vi "cluster to global variables.vi"(11 "Input Variables and Slopes in":T1 {"Height of Sample Box" format="%.2f"; "Reservoir Pressure" format="%.2f"; "Flow Offset" format="%.2f"; "String Pot Offset" format="%.2f"; "Aux 3 Offset" format="%.2f"; "Aux 2 Offset" format="%.2f"; "Aux 1 Offset" format="%.2f"; "Aux 3 Slope" format="%.2f"; "Aux 2 Slope" format="%.2f"; "Aux 1 Slope" format="%.2f"; "Up Hole  Pressure Offset" format="%.2f"; "DH Pressure Offset" format="%.2f"; "DH Pressure Trans Slope" format="%.2f"; "Atmospheric Pressure" format="%.2f"; "Depth to Water Table" format="%.2f"; "Up Hole Pressure Slope" format="%.2f"; "Flow Slope" format="%.2f"; "String Pot Slope" format="%.2f"; "Total Volume" format="%.2f"}) -> ()   [LabVIEW 2016]
uses:
  KPRO_2016 subvis/Control 2.ctl
  KPRO_2016 subvis/Kpro Globals.vi
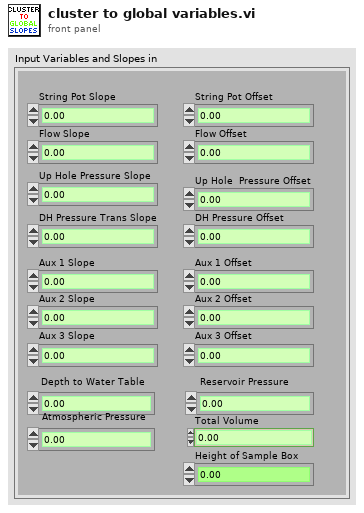
[diagram p1: front panel]
types:
  T1 = typedef "Control 2.ctl" = cluster{"Total Volume":dbl, "String Pot Slope":dbl, "Flow Slope":dbl, "Up Hole Pressure Slope":dbl, "Depth to Water Table":dbl, "Atmospheric Pressure":dbl, "DH Pressure Trans Slope":dbl, "DH Pressure Offset":dbl, "Up Hole  Pressure Offset":dbl, "Aux 1 Slope":dbl, "Aux 2 Slope":dbl, "Aux 3 Slope":dbl, "Aux 1 Offset":dbl, "Aux 2 Offset":dbl, "Aux 3 Offset":dbl, "String Pot Offset":dbl, "Flow Offset":dbl, "Reservoir Pressure":dbl, "Height of Sample Box":dbl}
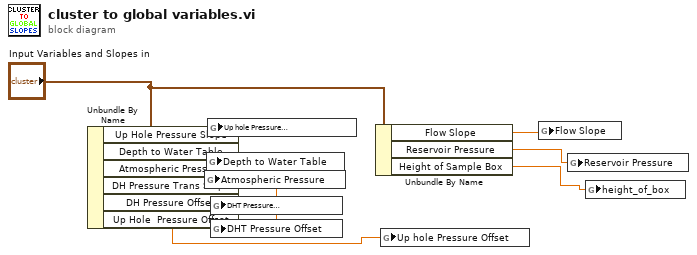
[diagram p0: block diagram]
diagram:
  n1 = Unbundle By Name("Input Variables and Slopes in") -> ("Up Hole Pressure Slope"=w1:dbl, "Depth to Water Table"=w2:dbl, "Atmospheric Pressure"=w3:dbl, "DH Pressure Trans Slope"=w4:dbl, "DH Pressure Offset"=w5:dbl, "Up Hole  Pressure Offset"=w6:dbl)
  n2 = global write "Kpro Globals.vi" "Atmospheric Pressure"(w3) -> ()
  n3 = global write "Kpro Globals.vi" "Depth to Water Table"(w2) -> ()
  n4 = global write "Kpro Globals.vi" "Up hole Pressure \nSlope"(w1) -> ()
  n5 = global write "Kpro Globals.vi" "DHT Pressure \nSlope"(w4) -> ()
  n6 = global write "Kpro Globals.vi" "DHT Pressure Offset"(w5) -> ()
  n7 = Unbundle By Name("Input Variables and Slopes in") -> ("Flow Slope"=w8:dbl, "Reservoir Pressure"=w9:dbl, "Height of Sample Box"=w10:dbl)
  n8 = global write "Kpro Globals.vi" "Up hole Pressure Offset"(w6) -> ()
  n9 = global write "Kpro Globals.vi" "Flow Slope"(w8) -> ()
  n10 = global write "Kpro Globals.vi" "Reservoir Pressure"(w9) -> ()
  n11 = global write "Kpro Globals.vi" "height_of_box"(w10) -> ()
